vi "update.vi"   [LabVIEW 2024]
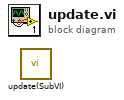
[diagram p0: block diagram]
diagram:
  n1 = call "update(SubVI).vi"() -> ()  [unwired: 9 in, 3 out]
